vi "KeyboardNanoDriveControl -SubVI.vi"() -> ()   [LabVIEW 2014]
uses:
  <vilib>/Utility/inputDevices.llb/keyboardAcquire.vi
  <vilib>/Utility/inputDevices.llb/closeKeyboard.vi
  <userlib>/Madlib/Madlib.dll
panel:
  in  "Command rate":u16(ring)=10 items=["500 Hertz"=2, "100 Hertz"=10, "10 Hertz"=100, "1 Hertz"=1000]
  in  "Motion Multiplier":dbl(slide)=9.904761904761905 scale=1.0..100.0
  in  "Max Velocity":string(combo)="22"
  in  "Z Decreasing":string(combo)="21"
  in  "Z Increasing":string(combo)="24"
  out "Z Calibration":dbl
  out "Y Calibration":dbl
  out "X Calibration":dbl
  out "Z Position":dbl format="%.3f"
  out "Y Position":dbl format="%.3f"
  out "X Position":dbl format="%.3f"
  in  "X Increasing":string(combo)="28"
  in  "X Decreasing":string(combo)="32"
  in  "Y Decreasing":string(combo)="10"
  in  "Y Increasing":string(combo)="13"
  out "First Key":T1(ring)
  in  "stop 2":bool
  # "Position Monitor"
  # "(um)"
  # "Max. Range"
  # "(um)"
  # "Options"
  # "Command Rate"
  # "Motion Multiplier"
  # "x1"
  # "x100"
  # "GamePad Key Configuration"
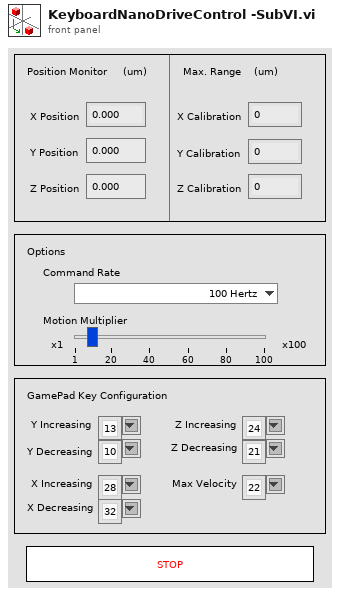
[diagram p1: front panel]
types:
  T1 = enum16{"0", "1", "2", "3", "4", "5", "6", "7", "8", "9", "A", "B", "C", "D", "E", "F", "G", "H", "I", "J", "K", "L", "M", "N", "O", "P", "Q", "R", "S", "T", "U", "V", "W", "X", "Y", "Z", "F1", "F2", "F3", "F4", "F5", "F6", "F7", "F8", "F9", "F10", "F11", "F12", "F13", "F14", "F15", "ADD", "BACK", "BACKSLASH", "CAPITAL", "COMMA", "DECIMAL", "DELETE", "DIVIDE", "DOWN", "END", "EQUALS", "ESCAPE", "GRAVE (`)", "HOME", "INSERT", "LBRACKET", "LCONTROL", "LEFT", "L ALT", "LSHIFT", "LWIN", "MINUS", "MULTIPLY", "NEXT", "NUMLOCK", "NUMPAD_0", "NUMPAD_1", "NUMPAD_2", "NUMPAD_3", "NUMPAD_4", "NUMPAD_5", "NUMPAD_6", "NUMPAD_7", "NUMPAD_8", "NUMPAD_9", "PAUSE", "PERIOD", "PRIOR (PG UP)", "RBRACKET", "RCONTROL", "RETURN", "RIGHT", "R ALT", "RSHIFT", "RWIN", "SCROLL", "SEMICOLON", "SLASH", "SPACE", "SUBTRACT", "TAB", "UP", "ENTER (num pad)", "' (quote)"}
  T2 = cluster{"X Command":dbl, "Y Command":dbl, "Z Command":dbl, "X Position":dbl, "Y Position":dbl, "Z Position":dbl, "X Calibration":dbl, "Y Calibration":dbl, "Z Calibration":dbl}
  T3 = cluster{"X Command":dbl, "Y Command":dbl, "Z Command":dbl, "X Position":dbl, "Y Position":dbl, "Z Position":dbl}
  T4 = enum16{"0", "1", "2", "3", "4", "5", "6", "7", "8", "9", "A", "B", "C", "D", "E", "F", "G", "H", "I", "J", "K", "L", "M", "N", "O", "P", "Q", "R", "S", "T", "U", "V", "W", "X", "Y", "Z", "F1", "F2", "F3", "F4", "F5", "F6", "F7", "F8", "F9", "F10", "F11", "F12", "F13", "F14", "F15", "ADD", "BACK", "BACKSLASH", "CAPITAL", "COMMA", "DECIMAL", "DELETE", "DIVIDE", "DOWN", "END", "EQUALS", "ESCAPE", "GRAVE (`)", "HOME", "INSERT", "LBRACKET", "LCONTROL", "LEFT", "L ALT", "LSHIFT", "LWIN", "MINUS", "MULTIPLY", "NEXT", "NUMLOCK", "NUMPAD_0", "NUMPAD_1", "NUMPAD_2", "NUMPAD_3", "NUMPAD_4", "NUMPAD_5", "NUMPAD_6", "NUMPAD_7", "NUMPAD_8", "NUMPAD_9", "PAUSE", "PERIOD", "PRIOR (PG UP)", "RBRACKET", "RCONTROL", "RETURN", "RIGHT", "R ALT", "RSHIFT", "RWIN", "SCROLL", "SEMICOLON", "SLASH", "SPACE", "SUBTRACT", "TAB", "UP", "ENTER (num pad)", "' (quote)"}[]
  T5 = cluster{"Y Increasing":string, "Y Decreasing":string, "X Decreasing":string, "X Increasing":string, "Z Increasing":string, "Z Decreasing":string, "Max Velocity":string}
  T6 = cluster{"X Command":dbl, "Y Command":dbl, "Pos. Command":dbl, "X Position":dbl, "Y Position":dbl, "position":dbl}
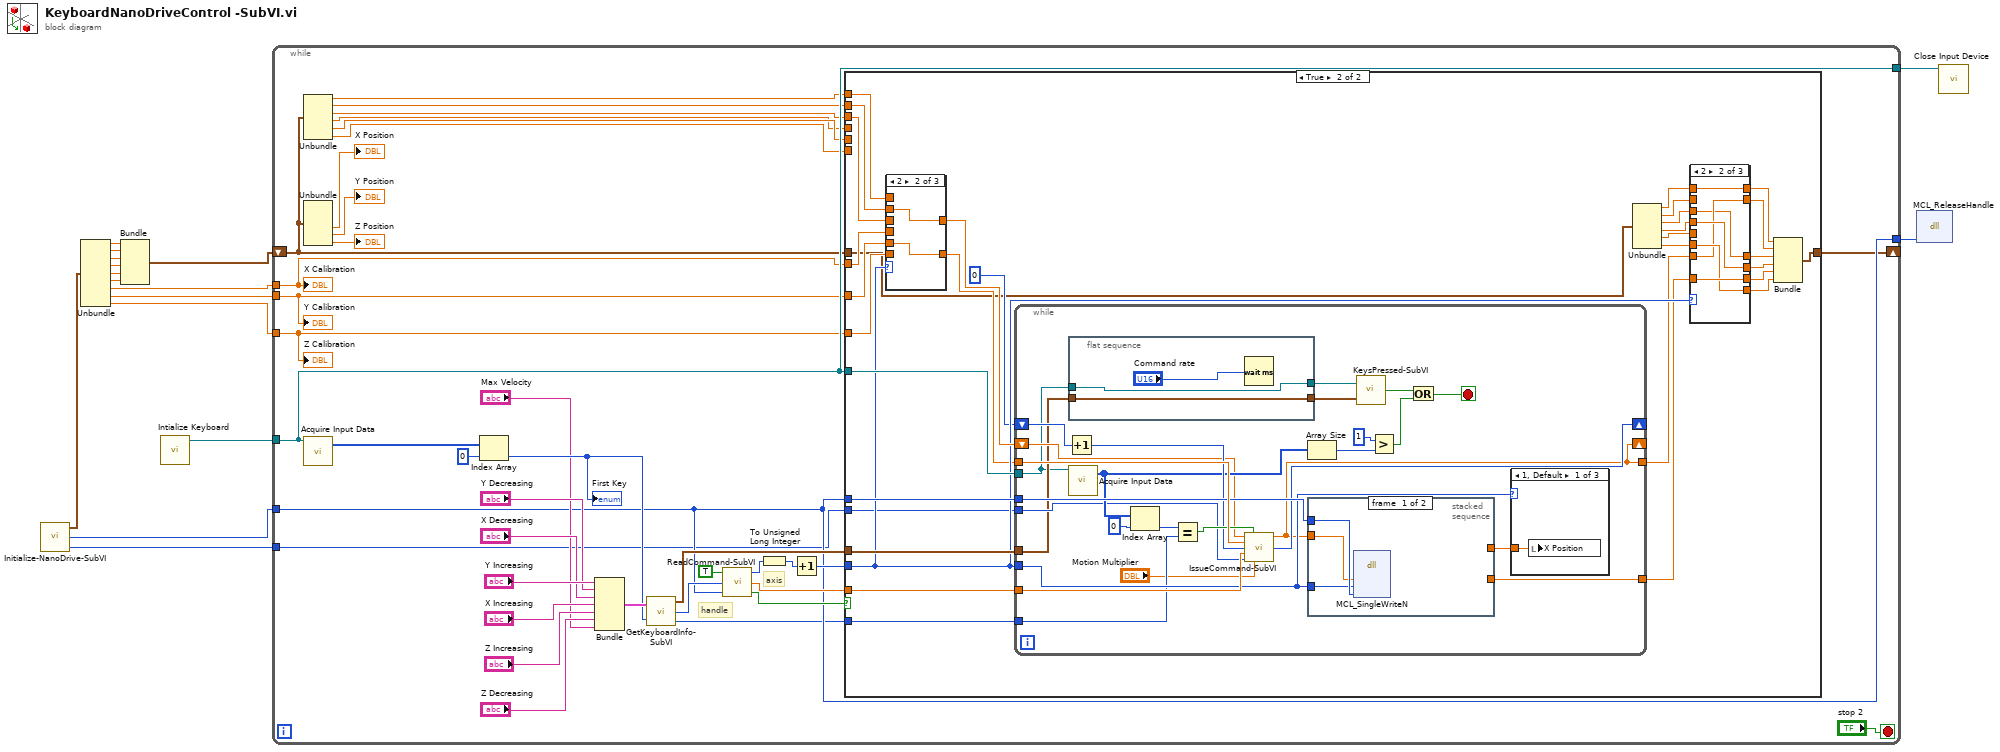
[diagram p0: block diagram]
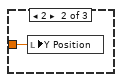
[diagram p7: hidden frame]
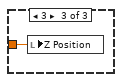
[diagram p8: hidden frame]
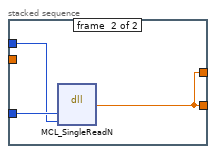
[diagram p9: hidden frame]
diagram:
  n1 = call <userlib>:"Initialize-NanoDrive-SubVI.vi"() -> ("Output Pos Info"=w13:T2, "Handle"=w12:i32, "ADC/DAC Resolution"=w11:u32)  [unwired: 1 out]
  n2 = Unbundle(w13) -> ("X Command"=w7:dbl, "Y Command"=w6:dbl, "Z Command"=w5:dbl, "X Position"=w4:dbl, "Y Position"=w3:dbl, "Z Position"=w2:dbl, "X Calibration"=w8:dbl, "Y Calibration"=w9:dbl, "Z Calibration"=w10:dbl)
  n3 = Bundle("X Command"=w7, "Y Command"=w6, "Z Command"=w5, "X Position"=w4, "Y Position"=w3, "Z Position"=w2) -> (w1:T3)  [unwired: 1 out]
  n4 = call <vilib>:"Intialize Keyboard.vi"() -> ("device ID"=w15:refnum<k1>)  [unwired: 1 in, 10 out]
  n5 = while {
    tunnel: w12 -> [w34]
    tunnel: [w34] -> w16
    tunnel: w15 -> [w30]
    tunnel: [w30] -> w14
    tunnel: w8 -> [w17]
    tunnel: w9 -> [w18]
    tunnel: w10 -> [w19]
    shift-right: [w32] -> _
    shift-left: w1 -> [w23]
    tunnel: w11 -> [w31]
    stop <- "stop 2" stop-if-true
    # "handle"
    # "axis"
    n6 = Unbundle(w23) -> ("X Command"=w24:dbl, "Y Command"=w25:dbl, "Z Command"=w26:dbl, "X Position"=w27:dbl, "Y Position"=w28:dbl, "Z Position"=w29:dbl)
    n7 = Unbundle(w23) -> ("X Position"=→"X Position":dbl, "Y Position"=→"Y Position":dbl, "Z Position"=→"Z Position":dbl)  [unwired: 3 out]
    n8 = call-poly <vilib>:"Acquire Input Data.vi"("device ID"=w30) -> ("keys pressed"=w52:T4)  [unwired: 1 in, 17 out]
    n9 = Index Array "Index Array"(array=w52, index=0) -> (element=w37:T1)
    "First Key" <- w37
    n10 = Bundle("Y Increasing"="Y Increasing", "Y Decreasing"="Y Decreasing", "X Decreasing"="X Decreasing", "X Increasing"="X Increasing", "Z Increasing"="Z Increasing", "Z Decreasing"="Z Decreasing", "Max Velocity"="Max Velocity") -> (w38:T5)  [unwired: 1 out]
    n11 = call <userlib>:"GetKeyboardInfo-SubVI.vi"("Key Selections"=w38, "Key\nValue"=w37) -> ("Key values"=w49:cluster{i32, i32, i32, i32, i32, i32, i32}, "number"=w51:u32, "Max Velocity Value"=w33:i32)
    n12 = call <userlib>:"ReadCommand-SubVI.vi"("handle"=w34, "Motion #"=w51, "Enable\n(True)"=TRUE ("JoyStick Option")) -> ("Enable Move\n(TRUE)"=w35:bool, "Direction"=w45:dbl, "Axis"=w48:enum16{"X", "Y", "Z"})
    n13 = To Unsigned Long Integer(number=w48) -> (unsigned 32bit integer=w47:u32)
    n14 = Increment(x=w47) -> (x+1=w46:u32)
    n15 = case shown="True" w35 {
      tunnel: w34 -> [_ w87]
      tunnel: w30 -> [_ w86]
      tunnel: w49 -> [_ w85]
      tunnel: w27 -> [_ _]
      tunnel: w28 -> [_ _]
      tunnel: w29 -> [_ _]
      tunnel: w46 -> [_ w83]
      tunnel: w45 -> [_ w81]
      tunnel: w17 -> [_ w80]
      tunnel: w18 -> [_ w79]
      tunnel: w19 -> [_ w78]
      tunnel: w33 -> [_ w75]
      tunnel: w23 -> [w55 w74]
      tunnel: [w55 w73] -> w32
      tunnel: w31 -> [_ w72]
      tunnel: w26 -> [_ w63]
      tunnel: w25 -> [_ w64]
      tunnel: w24 -> [_ w65]
      frame False {
      }
      frame True {
        n16 = case shown="2" w83 {
          tunnel: w65 -> [w107 _ _]
          tunnel: w64 -> [_ w109 _]
          tunnel: w63 -> [_ _ w111]
          tunnel: [w107 w109 w111] -> w84
          tunnel: w80 -> [w106 _ _]
          tunnel: w79 -> [_ w108 _]
          tunnel: w78 -> [_ _ w110]
          tunnel: [w106 w108 w110] -> w77
          frame 1, Default {
          }
          frame 2 {
          }
          frame 3 {
          }
        }
        n17 = while {
          tunnel: w87 -> [w134]
          tunnel: w86 -> [w112]
          tunnel: w85 -> [w114]
          tunnel: w83 -> [w133]
          tunnel: [w137] -> w82
          tunnel: w81 -> [w136]
          tunnel: w77 -> [w135]
          shift-right: [w116] -> _
          shift-left: w84 -> [w117]
          shift-right: [w126] -> _
          shift-left: 0 -> [w128]
          tunnel: w75 -> [w125]
          tunnel: w72 -> [w118]
          tunnel: [w116] -> w62
          stop <- w124 stop-if-true
          n18 = Increment(x=w128) -> (x+1=w127:i32)
          n19 = flat-sequence {
            tunnel: [w140] -> w115
            tunnel: w112 -> [w140]
            tunnel: [w139] -> w113
            tunnel: w114 -> [w139]
            frame #0 {
              n20 = Wait (ms)(milliseconds to wait="Command rate") -> ()  [unwired: 1 out]
            }
          }
          n21 = call-poly <vilib>:"Acquire Input Data.vi"("device ID"=w112) -> ("keys pressed"=w120:T4)  [unwired: 1 in, 17 out]
          n22 = Index Array(array=w120, index=0) -> (element=w131:T1)
          n23 = Equal?(x=w131, y=w125) -> (x = y?=w130:bool)
          n24 = call <userlib>:"IssueCommand-SubVI.vi"("Current Position"=w117, "Max Velocity?"=w130, "Calibration"=w135, "Loop Iteration"=w127, "Direction"=w136, "ADC/DAC Resolution"=w118, "Motion Multiplier"="Motion Multiplier") -> ("Pos. Command"=w116:dbl, "Loop Iteration Out"=w126:i32)  [unwired: 7 out]
          n25 = Array Size(array=w120) -> (size(s)=w122:i32)
          n26 = stacked-sequence {
            tunnel: w134 -> [w147 w149]
            tunnel: w133 -> [w146 w150]
            tunnel: [_ w148] -> w137
            tunnel: w116 -> [w145 _]
            tunnel: [_ w148] -> w129
            frame #0 {
              n27 = dll-call lib="C:/Program Files (x86)/National Instruments/LabVIEW 2014/user.lib/Madlib/Madlib.dll" fn="MCL_SingleWriteN" label="Madlib.dll\nMCL_SingWriteN"("position"=w145, "axis"=w146, "handle"=w147) -> ()  [unwired: 6 in, 3 out]
            }
            frame #1 {
              n28 = dll-call lib="C:/Program Files (x86)/National Instruments/LabVIEW 2014/user.lib/Madlib/Madlib.dll" fn="MCL_SingleReadN" label="Madlib.dll:\nMCL_SingleReadN"("Axis"=w150, "Handle"=w149) -> ("position"=w148:dbl)  [unwired: 5 in, 2 out]
            }
          }
          n29 = call <userlib>:"KeysPressed-SubVI.vi"("Key values"=w113, "device ID"=w115) -> ("Stop = TRUE"=w138:bool)
          n30 = Greater?(x=1, y=w122) -> (0:w123:bool)
          n31 = Or(x=w138, y=w123) -> (x .or. y?=w124:bool)
          n32 = case shown="1, Default" w133 {
            tunnel: w129 -> [w142 w143 w144]
            frame 1, Default {
              n33 = local write "X Position"(w142) -> ()
            }
            frame 2 {
              n34 = local write "Y Position"(w143) -> ()
            }
            frame 3 {
              n35 = local write "Z Position"(w144) -> ()
            }
          }
        }
        n36 = Unbundle(w74) -> ("X Command"=w61:dbl, "Y Command"=w60:dbl, "Z Command"=w59:dbl, "X Position"=w71:dbl, "Y Position"=w70:dbl, "Z Position"=w69:dbl)
        n37 = case shown="2" w83 {
          tunnel: w71 -> [_ w98 w104]
          tunnel: w70 -> [w93 _ w103]
          tunnel: w69 -> [w92 w97 _]
          tunnel: w82 -> [w91 w99 w105]
          tunnel: [w91 w98 w104] -> w66
          tunnel: [w93 w99 w103] -> w67
          tunnel: [w92 w97 w105] -> w68
          tunnel: w62 -> [w90 w96 w100]
          tunnel: w61 -> [_ w95 w102]
          tunnel: w60 -> [w89 _ w101]
          tunnel: w59 -> [w88 w94 _]
          tunnel: [w90 w95 w102] -> w56
          tunnel: [w89 w96 w101] -> w57
          tunnel: [w88 w94 w100] -> w58
          frame 1, Default {
          }
          frame 2 {
          }
          frame 3 {
          }
        }
        n38 = Bundle("X Command"=w56, "Y Command"=w57, "Pos. Command"=w58, "X Position"=w66, "Y Position"=w67, "position"=w68) -> (w73:T6)  [unwired: 1 out]
      }
    }
    "X Calibration" <- w17
    "Y Calibration" <- w18
    "Z Calibration" <- w19
  }
  n39 = dll-call lib="C:/Program Files (x86)/National Instruments/LabVIEW 2014/user.lib/Madlib/Madlib.dll" fn="MCL_ReleaseHandle" label="Madlib.dll:\nMCL_ReleaseHandle"("handle"=w16) -> ()  [unwired: 4 in, 3 out]
  n40 = call-poly <vilib>:"Close Input Device.vi"("device ID"=w14) -> ()  [unwired: 1 in, 9 out]
